vi "GUI Close Synchronization Objects.vi"(8 "error in (no error)":errorcluster, 11 "FOFB GUI":T1) -> (0 "error out":errorcluster)   [LabVIEW 2011, in "User Interface VIs.lvlib"]
uses:
  User Interface VIs.lvlib
  Types Definitions/Type FOFB GUI.ctl
  Types Definitions/Type Configuration Data (GUI to Controller).ctl
  Types Definitions/Type Monitoring Data.ctl
  Types Definitions/Type Diagnostics Data.ctl
  Types Definitions/Type CPU Loads Array.ctl
  Types Definitions/Type CPU Loads.ctl
  Types Definitions/Type Diagnostics Sample.ctl
  Types Definitions/Type Monitoring Sample.ctl
  Type Definitions.lvlib
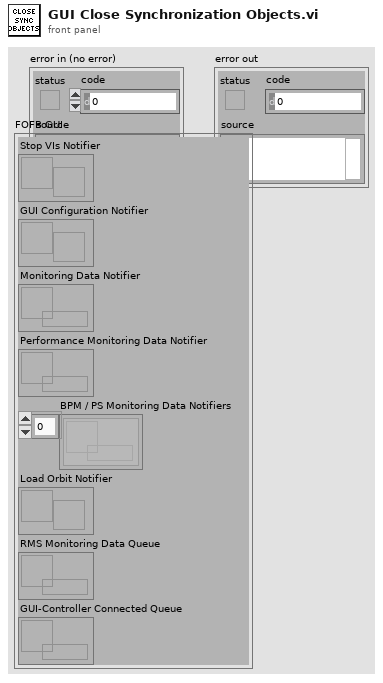
[diagram p1: front panel]
types:
  T1 = typedef "Type Definitions.lvlib/Type FOFB GUI.ctl" = cluster{"Stop VIs Notifier":refnum<notifier>, "GUI Configuration Notifier":refnum<notifier>, "Monitoring Data Notifier":refnum<queue>, "Performance Monitoring Data Notifier":refnum<queue>, "BPM / PS Monitoring Data Notifiers":refnum<queue>[], "Load Orbit Notifier":refnum<notifier>, "RMS Monitoring Data Queue":refnum<queue>, "GUI-Controller Connected Queue":refnum<queue>}
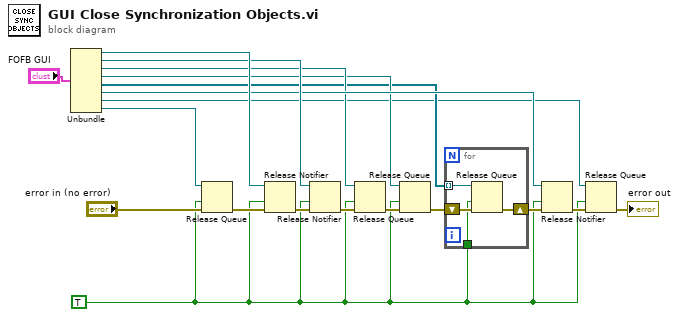
[diagram p0: block diagram]
diagram:
  w1 = TRUE ("force destroy? (F)")
  n1 = Unbundle("FOFB GUI") -> ("Stop VIs Notifier"=w18:refnum<notifier>, "GUI Configuration Notifier"=w17:refnum<notifier>, "Monitoring Data Notifier"=w15:refnum<queue>, "Performance Monitoring Data Notifier"=w14:refnum<queue>, "BPM / PS Monitoring Data Notifiers"=w13:refnum<queue>[], "Load Orbit Notifier"=w16:refnum<notifier>, "RMS Monitoring Data Queue"=w7:refnum<queue>, "GUI-Controller Connected Queue"=w2:refnum<queue>)
  n2 = Release Queue(queue=w2, force destroy? (F)=w1, error in (no error)="error in (no error)") -> (error out=w3:errorcluster)  [unwired: 2 out]
  n3 = Release Notifier(notifier=w18, force destroy? (F)=w1, error in (no error)=w3) -> (error out=w12:errorcluster)  [unwired: 2 out]
  n4 = Release Notifier(notifier=w17, force destroy? (F)=w1, error in (no error)=w12) -> (error out=w11:errorcluster)  [unwired: 2 out]
  n5 = Release Queue(queue=w15, force destroy? (F)=w1, error in (no error)=w11) -> (error out=w10:errorcluster)  [unwired: 2 out]
  n6 = Release Queue(queue=w14, force destroy? (F)=w1, error in (no error)=w10) -> (error out=w9:errorcluster)  [unwired: 2 out]
  n7 = for {
    tunnel: w13 -> [w23] mode=indexing
    shift-right: [w21] -> w8
    shift-left: w9 -> [w22]
    tunnel: w1 -> [w20]
    n8 = Release Queue(queue=w23, force destroy? (F)=w20, error in (no error)=w22) -> (error out=w21:errorcluster)  [unwired: 2 out]
  }
  n9 = Release Notifier(notifier=w16, force destroy? (F)=w1, error in (no error)=w8) -> (error out=w6:errorcluster)  [unwired: 2 out]
  n10 = Release Queue(queue=w7, force destroy? (F)=w1, error in (no error)=w6) -> (error out=→"error out":errorcluster)  [unwired: 2 out]
